vi "BackTrackingAstar.vi"() -> ()   [LabVIEW 2016]
uses:
  CameFrom.ctl
panel:
  in  "CameFrom":T1
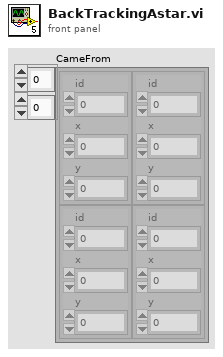
[diagram p1: front panel]
types:
  T1 = typedef "CameFrom.ctl" = cluster{"id":dbl, "x":dbl, "y":dbl}[][]
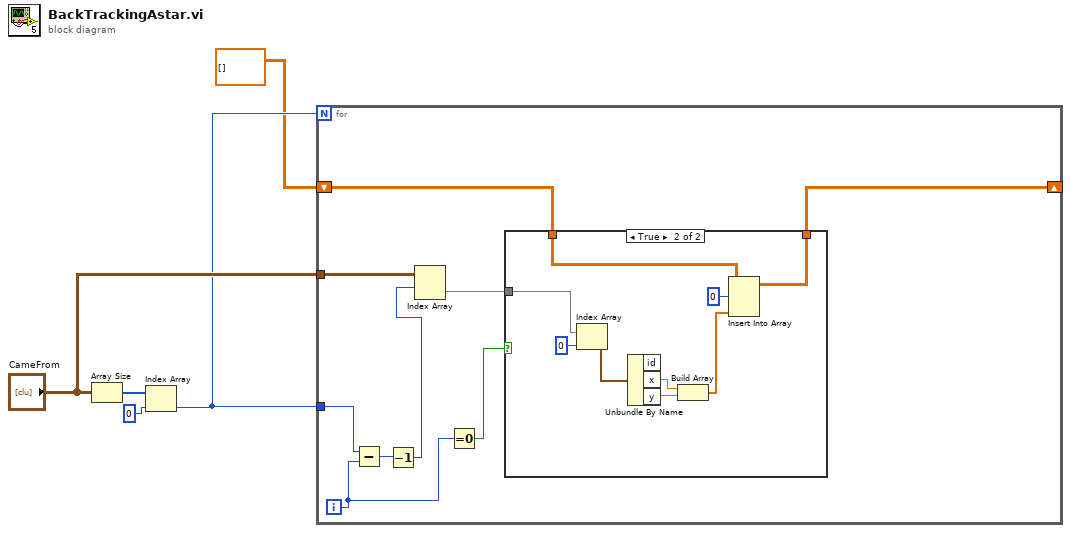
[diagram p0: block diagram]
diagram:
  n1 = Array Size(array="CameFrom") -> (size(s)=w5:i32[])
  n2 = Index Array(array=w5, index=0) -> (element=w2:i32)
  n3 = for {
    N: w2 -> [_]
    tunnel: "CameFrom" -> [w11]
    tunnel: w2 -> [w14]
    shift-right: [w6] -> _
    shift-left: dbl[][] [] ("Path") -> [w7]
    i -> [w10]
    n4 = Subtract(x=w14, y=w10) -> (x-y=w13:i32)
    n5 = Decrement(x=w13) -> (x-1=w12:i32)
    n6 = Index Array(array=w11, index (row)=w12) -> (element=w8:cluster{"id":dbl, "x":dbl, "y":dbl}[])  [unwired: 1 in]
    n7 = Equal To 0?(x=w10) -> (x = 0?=w9:bool)
    n8 = case shown="True" w9 {
      tunnel: w8 -> [_ w19]
      tunnel: w7 -> [_ w18]
      tunnel: [_ w15] -> w6
      frame False {
      }
      frame True {
        n9 = Index Array(array=w19, index=0) -> (element=w22:cluster{"id":dbl, "x":dbl, "y":dbl})
        n10 = Unbundle By Name(w22) -> ("x"=w21:dbl, "y"=w20:dbl)  [unwired: 1 out]
        n11 = Build Array(w21, w20) -> (w17:dbl[])
        n12 = Insert Into Array(array=w18, index (row)=0, new element=w17) -> (w15:dbl[][])  [unwired: 1 in]
      }
    }
  }
